vi "LDA1_Safety.vi"(1 "Adam Loop Count":i32, 2 "Ch Names":string[](array[string]), 3 "Values":dbl[](array[numeric]) format="%.2f") -> (0 "Scan comment":string)   [LabVIEW 2013]
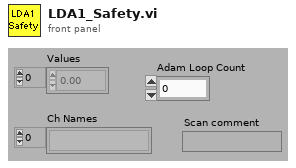
[diagram p1: front panel]
types:
  T1 = typedef "LVDateTimeRec.ctl" = cluster{"fractional second":dbl, "second":i32, "minute":i32, "hour":i32, "day of month":i32, "month":i32, "year":i32, "day of week":i32, "day of year":i32, "DST":i32}
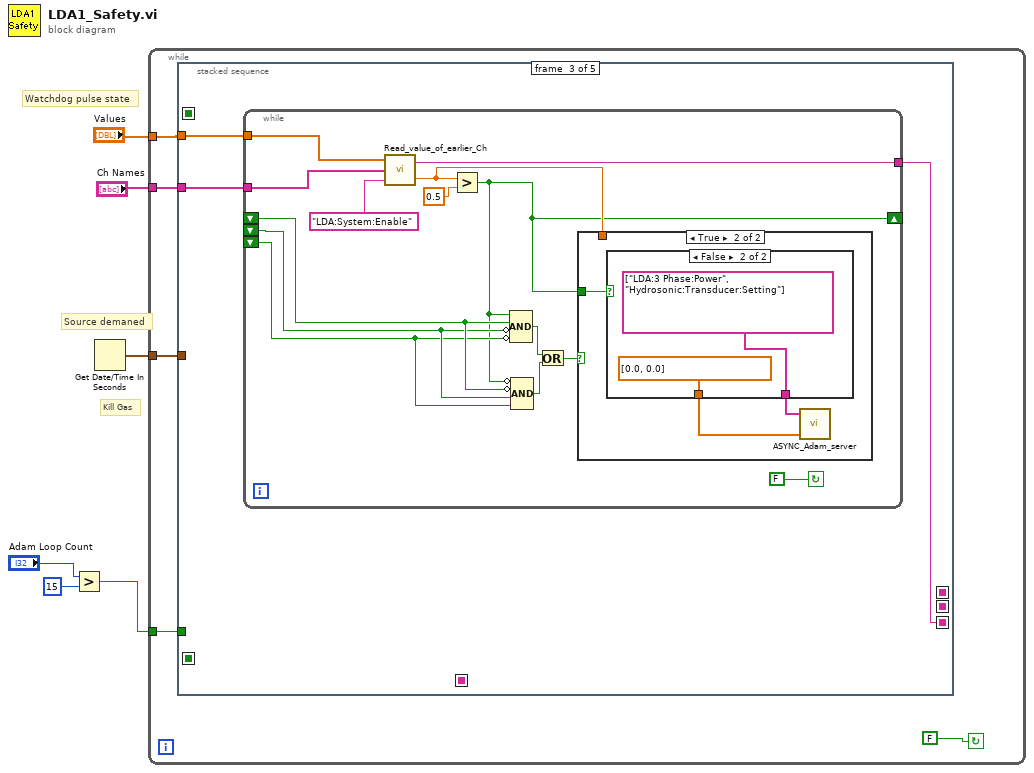
[diagram p0: block diagram]
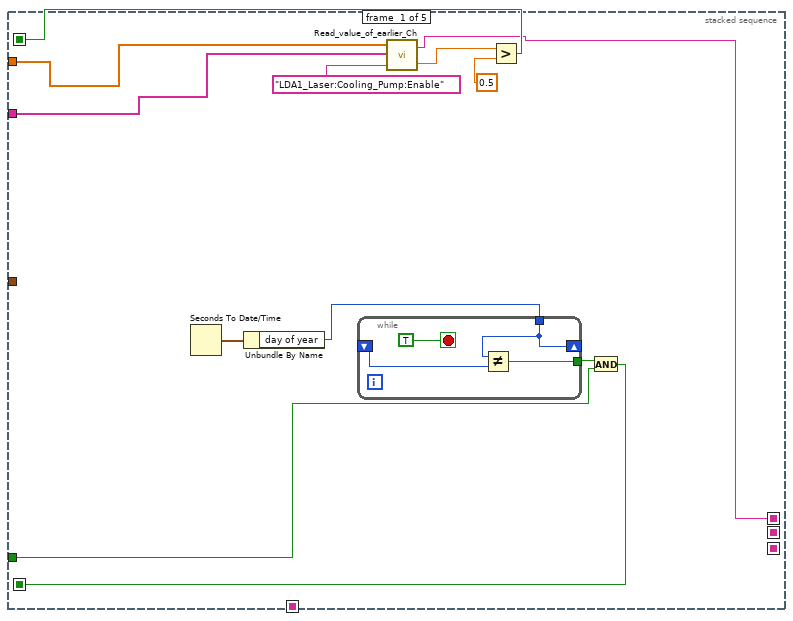
[diagram p2: hidden frame]
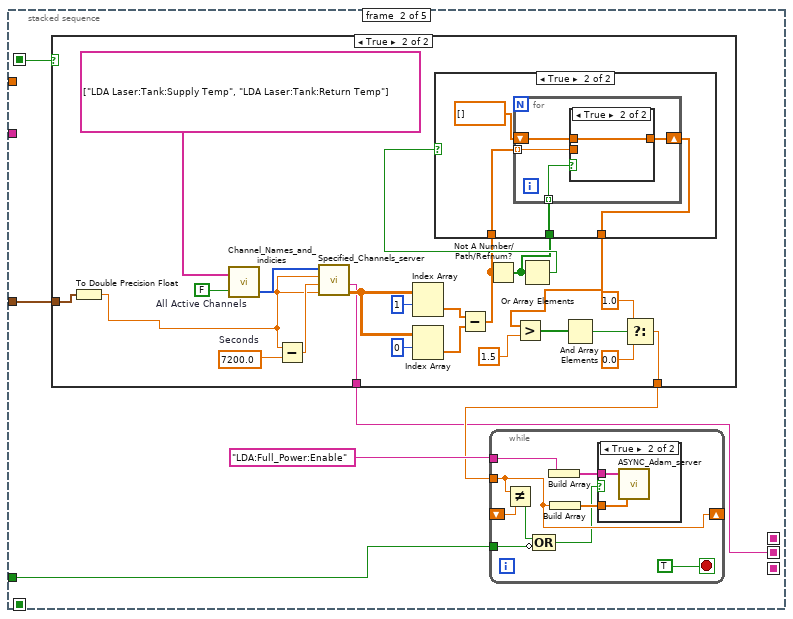
[diagram p3: hidden frame]
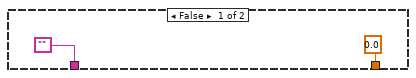
[diagram p5: hidden frame]
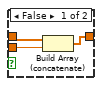
[diagram p7: hidden frame]
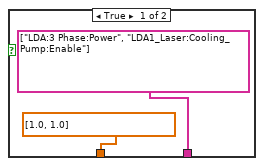
[diagram p9: hidden frame]
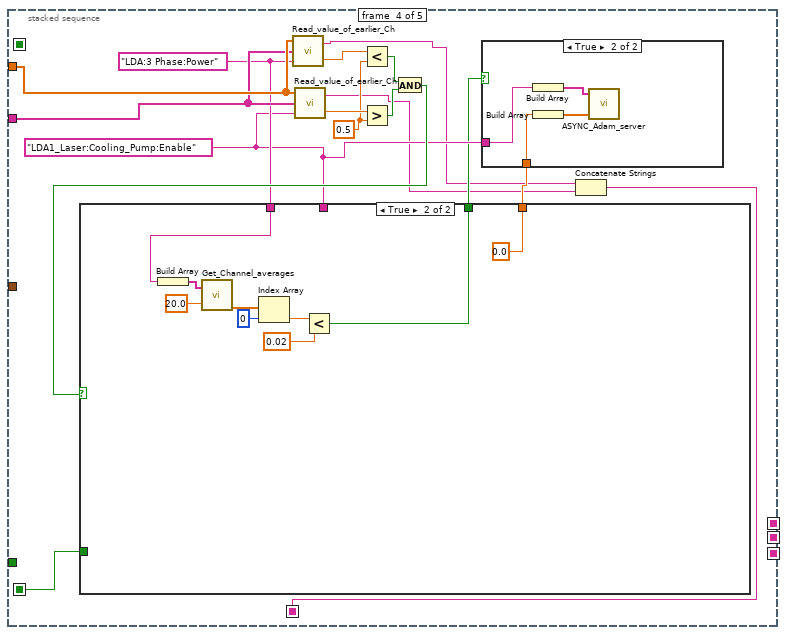
[diagram p10: hidden frame]
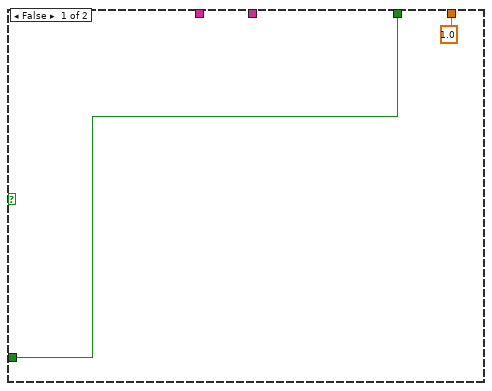
[diagram p12: hidden frame]
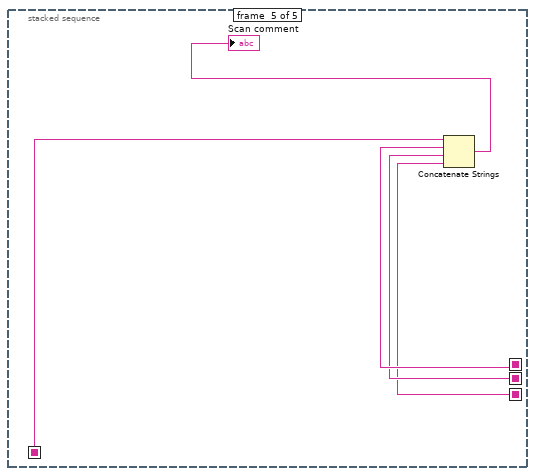
[diagram p13: hidden frame]
diagram:
  # "Source demaned"
  # "Watchdog pulse state"
  # "Kill Gas"
  n1 = Greater?(x="Adam Loop Count", y=15) -> (0:w2:bool)
  n2 = Get Date/Time In Seconds() -> (seconds since 1Jan1904=w1:timestamp)
  n3 = while {
    tunnel: "Ch Names" -> [w11]
    tunnel: "Values" -> [w10]
    tunnel: w2 -> [w8]
    tunnel: w1 -> [w7]
    stop <- FALSE continue-if-true
    n4 = stacked-sequence {
      seq-local: [w13 _ _ _ _] -> [_ _ _ w110 _]
      seq-local: [w21 _ _ _ _] -> [_ w32 _ _ _]
      seq-local: [w17 _ _ _ _] -> [_ _ _ _ w142]
      seq-local: [_ w28 _ _ _] -> [_ _ _ _ w141]
      seq-local: [_ _ w83 _ _] -> [_ _ _ _ w140]
      seq-local: [_ _ _ w107 _] -> [_ _ _ _ w138]
      tunnel: w11 -> [w22 _ w84 w120 _]
      tunnel: w10 -> [w23 _ w85 w121 _]
      tunnel: w8 -> [w12 w30 _ _ _]
      tunnel: w7 -> [_ w33 _ _ _]
      frame #0 {
        n5 = Seconds To Date/Time() -> (date time rec=w16:T1)  [unwired: 2 in]
        n6 = Unbundle By Name(w16) -> ("day of year"=w15:i32)
        n7 = while {
          shift-right: [w27] -> _
          shift-left: _ -> [w26]
          tunnel: w15 -> [w27]
          tunnel: [w25] -> w14
          stop <- TRUE stop-if-true
          n8 = Not Equal?(x=w27, y=w26) -> (x != y?=w25:bool)
        }
        n9 = call "Read_value_of_earlier_Ch.vi"("Desired Ch to Read"="LDA1_Laser:Cooling_Pump:Enable", "Ch names"=w22, "Present scan array"=w23) -> ("Value"=w19:dbl, "Scan comment"=w17:string)  [unwired: 1 in]
        n10 = Greater?(x=w19, y=0.5) -> (0:w21:bool)
        n11 = And(x=w14, y=w12) -> (x .and. y?=w13:bool)
      }
      frame #1 {
        n12 = case shown="True" w32 {
          tunnel: w33 -> [_ w69]
          tunnel: [0.0 ("y") w54] -> w29
          tunnel: ["" w47] -> w28
          frame False {
          }
          frame True {
            w67 = 7200.0  # Seconds
            w65 = FALSE  # All Active Channels
            n13 = To Double Precision Float(number=w69) -> (double precision float=w63:dbl)
            n14 = call "Channel_Names_and_indicies.vi"("All Active Channels"=w65, "Desired Ch Names"=string[] ["LDA Laser:Tank:Supply Temp", "LDA Laser:Tank:Return Temp"]) -> ("Indicies"=w66:i32[])  [unwired: 1 out]
            n15 = Subtract(x=w63, y=w67) -> (x-y=w68:dbl)
            n16 = call "Specified_Channels_server.vi"("End time"=w63, "Start time"=w68, "Clients time"=w63, "Requested channels"=w66) -> ("Output array"=w60:dbl[][], "Messages"=w47:string)  [unwired: 1 in, 3 out]
            n17 = Index Array(array=w60, index (row)=1) -> (element=w59:dbl[])  [unwired: 1 in]
            n18 = Index Array(array=w60, index (row)=0) -> (element=w58:dbl[])  [unwired: 1 in]
            n19 = Subtract(x=w59, y=w58) -> (x-y=w49:dbl[])
            n20 = Not A Number/Path/Refnum?(number/path/refnum=w49) -> (NaN/Path/Refnum?=w50:bool[])
            n21 = Or Array Elements(Boolean array=w50) -> (logical OR=w51:bool)
            n22 = case shown="True" w51 {
              tunnel: w50 -> [_ w74]
              tunnel: w49 -> [w70 w73]
              tunnel: [w70 w71] -> w48
              frame False {
              }
              frame True {
                n23 = for {
                  shift-right: [w77] -> w71
                  shift-left: dbl[] [] -> [w76]
                  tunnel: w74 -> [w78] mode=indexing
                  tunnel: w73 -> [w75] mode=indexing
                  n24 = case shown="True" w78 {
                    tunnel: [w80 w82] -> w77
                    tunnel: w76 -> [w81 w82]
                    tunnel: w75 -> [w79 _]
                    frame False {
                      n25 = Build Array (concatenate)(w81, w79) -> (w80:dbl[])
                    }
                    frame True {
                    }
                  }
                }
              }
            }
            n26 = Greater?(x=w48, y=1.5) -> (0:w53:bool[])
            n27 = And Array Elements(Boolean array=w53) -> (logical AND=w52:bool)
            n28 = Select(t=1.0 ("y"), s=w52, f=0.0 ("y")) -> (s? t:f=w54:dbl)
          }
        }
        n29 = while {
          shift-right: [w38] -> _
          shift-left: _ -> [w39]
          tunnel: w29 -> [w38]
          tunnel: "LDA:Full_Power:Enable" -> [w40]
          tunnel: w30 -> [w35]
          stop <- TRUE stop-if-true
          n30 = Not Equal?(x=w38, y=w39) -> (x != y?=w36:bool)
          n31 = Compound Arithmetic op=OR(w36, invert w35) -> (w34:bool)
          n32 = Build Array(w40) -> (w41:string[])
          n33 = Build Array(w38) -> (w42:dbl[])
          n34 = case shown="True" w34 {
            tunnel: w42 -> [_ w44]
            tunnel: w41 -> [_ w43]
            frame False {
            }
            frame True {
              n35 = call "ASYNC_Adam_server.vi"("Values"=w44, "Channel Names"=w43) -> ()  [unwired: 1 in, 3 out]
            }
          }
        }
      }
      frame #2 {
        n36 = while {
          tunnel: w85 -> [w99]
          tunnel: w84 -> [w98]
          shift-right: [w87] -> _
          shift-left: _ -> [w93]
          shift-left: _ -> [w92]
          shift-left: _ -> [w91]
          tunnel: [w86] -> w83
          stop <- FALSE continue-if-true
          n37 = call "Read_value_of_earlier_Ch.vi"("Desired Ch to Read"="LDA:System:Enable", "Ch names"=w98, "Present scan array"=w99) -> ("Value"=w94:dbl, "Scan comment"=w86:string)  [unwired: 1 in]
          n38 = Greater?(x=w94, y=0.5) -> (0:w87:bool)
          n39 = Compound Arithmetic op=AND(w87, w93, invert w92, invert w91) -> (w89:bool)
          n40 = Compound Arithmetic op=AND(invert w87, invert w93, w92, w91) -> (w90:bool)
          n41 = Or(x=w89, y=w90) -> (x .or. y?=w88:bool)
          n42 = case shown="True" w88 {
            tunnel: w94 -> [_ _]
            tunnel: w87 -> [_ w102]
            frame False {
            }
            frame True {
              n43 = case shown="False" w102 {
                tunnel: [string[] ["LDA:3 Phase:Power", "LDA1_Laser:Cooling_Pump:Enable"] ("Channel Names") string[] ["LDA:3 Phase:Power", "Hydrosonic:Transducer:Setting"] ("Channel Names")] -> w101
                tunnel: [dbl[] [1.0, 1.0] ("Values") dbl[] [0.0, 0.0] ("Values")] -> w100
                frame True {
                }
                frame False {
                }
              }
              n44 = call "ASYNC_Adam_server.vi"("Values"=w100, "Channel Names"=w101) -> ()  [unwired: 1 in, 3 out]
            }
          }
        }
      }
      frame #3 {
        w114 = "LDA:3 Phase:Power" ("Desired Ch to Read")
        w119 = 0.5 ("y")
        w113 = "LDA1_Laser:Cooling_Pump:Enable" ("Desired Ch to Read")
        n45 = call "Read_value_of_earlier_Ch.vi"("Desired Ch to Read"=w114, "Ch names"=w120, "Present scan array"=w121) -> ("Value"=w118:dbl, "Scan comment"=w109:string)  [unwired: 1 in]
        n46 = call "Read_value_of_earlier_Ch.vi"("Desired Ch to Read"=w113, "Ch names"=w120, "Present scan array"=w121) -> ("Value"=w122:dbl, "Scan comment"=w108:string)  [unwired: 1 in]
        n47 = Less?(x=w118, y=w119) -> (x < y?=w117:bool)
        n48 = Greater?(x=w122, y=w119) -> (0:w116:bool)
        n49 = And(x=w117, y=w116) -> (x .and. y?=w115:bool)
        n50 = case shown="True" w115 {
          tunnel: w114 -> [_ w131]
          tunnel: w113 -> [_ _]
          tunnel: [w127 w130] -> w112
          tunnel: [1.0 ("element") 0.0 ("element")] -> w111
          tunnel: w110 -> [w127 _]
          frame False {
          }
          frame True {
            n51 = Build Array(w131) -> (w136:string[])
            n52 = call "Get_Channel_averages.vi"("Desired Ch Names"=w136, "Averaging time (mins)"=20.0) -> ("number"=w135:dbl[])  [unwired: 1 in, 2 out]
            n53 = Index Array(array=w135, index=0) -> (element=w133:dbl)
            n54 = Less?(x=w133, y=0.02) -> (x < y?=w130:bool)
          }
        }
        n55 = case shown="True" w112 {
          tunnel: w113 -> [_ w124]
          tunnel: w111 -> [_ w123]
          frame False {
          }
          frame True {
            n56 = Build Array(w124) -> (w125:string[])
            n57 = Build Array(w123) -> (w126:dbl[])
            n58 = call "ASYNC_Adam_server.vi"("Values"=w126, "Channel Names"=w125) -> ()  [unwired: 1 in, 3 out]
          }
        }
        n59 = Concatenate Strings(w109, w108) -> (w107:string)
      }
      frame #4 {
        n60 = Concatenate Strings(w138, w142, w141, w140) -> (→"Scan comment":string)
      }
    }
  }
